vi "Read Global Message Count.vi"(8 "error in":errorcluster, 11 "Module Handle":u32) -> (0 "error out":errorcluster, 2 "Global Message Count":u32, 3 "Module Handle out":u32)   [LabVIEW 2020, in "AIM MIL-STD-1553 Hardware API.lvlib"]
uses:
  AIM MIL-STD-1553 Hardware API.lvlib
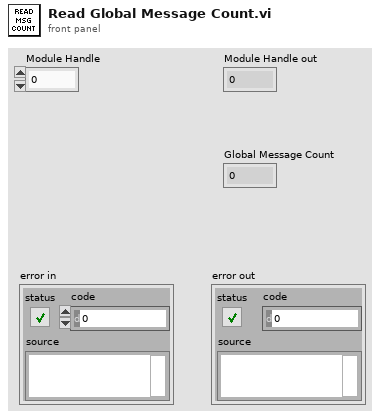
[diagram p1: front panel]
types:
  T1 = typedef "1553 All Status Counters.ctl" = cluster{"Global Message Count":u32, "Global Error Count":u32, "Primary Current Load":dbl, "Primary Average Load":dbl, "Secondary Current Load":dbl, "Secondary Average Load":dbl, "RT 1":cluster{"Active":bool, "Errors":bool, "Message Count":u32, "Error Count":u32}, "RT 2":cluster{"Active":bool, "Errors":bool, "Message Count":u32, "Error Count":u32}, "RT 3":cluster{"Active":bool, "Errors":bool, "Message Count":u32, "Error Count":u32}, "RT 4":cluster{"Active":bool, "Errors":bool, "Message Count":u32, "Error Count":u32}, "RT 5":cluster{"Active":bool, "Errors":bool, "Message Count":u32, "Error Count":u32}, "RT 6":cluster{"Active":bool, "Errors":bool, "Message Count":u32, "Error Count":u32}, "RT 7":cluster{"Active":bool, "Errors":bool, "Message Count":u32, "Error Count":u32}, "RT 8":cluster{"Active":bool, "Errors":bool, "Message Count":u32, "Error Count":u32}, "RT 9":cluster{"Active":bool, "Errors":bool, "Message Count":u32, "Error Count":u32}, "RT 10":cluster{"Active":bool, "Errors":bool, "Message Count":u32, "Error Count":u32}, "RT 11":cluster{"Active":bool, "Errors":bool, "Message Count":u32, "Error Count":u32}, "RT 12":cluster{"Active":bool, "Errors":bool, "Message Count":u32, "Error Count":u32}, "RT 13":cluster{"Active":bool, "Errors":bool, "Message Count":u32, "Error Count":u32}, "RT 14":cluster{"Active":bool, "Errors":bool, "Message Count":u32, "Error Count":u32}, "RT 15":cluster{"Active":bool, "Errors":bool, "Message Count":u32, "Error Count":u32}, "RT 16":cluster{"Active":bool, "Errors":bool, "Message Count":u32, "Error Count":u32}, "RT 17":cluster{"Active":bool, "Errors":bool, "Message Count":u32, "Error Count":u32}, "RT 18":cluster{"Active":bool, "Errors":bool, "Message Count":u32, "Error Count":u32}, "RT 19":cluster{"Active":bool, "Errors":bool, "Message Count":u32, "Error Count":u32}, "RT 20":cluster{"Active":bool, "Errors":bool, "Message Count":u32, "Error Count":u32}, "RT 21":cluster{"Active":bool, "Errors":bool, "Message Count":u32, "Error Count":u32}, "RT 22":cluster{"Active":bool, "Errors":bool, "Message Count":u32, "Error Count":u32}, "RT 23":cluster{"Active":bool, "Errors":bool, "Message Count":u32, "Error Count":u32}, "RT 24":cluster{"Active":bool, "Errors":bool, "Message Count":u32, "Error Count":u32}, "RT 25":cluster{"Active":bool, "Errors":bool, "Message Count":u32, "Error Count":u32}, "RT 26":cluster{"Active":bool, "Errors":bool, "Message Count":u32, "Error Count":u32}, "RT 27":cluster{"Active":bool, "Errors":bool, "Message Count":u32, "Error Count":u32}, "RT 28":cluster{"Active":bool, "Errors":bool, "Message Count":u32, "Error Count":u32}, "RT 29":cluster{"Active":bool, "Errors":bool, "Message Count":u32, "Error Count":u32}, "RT 30":cluster{"Active":bool, "Errors":bool, "Message Count":u32, "Error Count":u32}, "RT 31":cluster{"Active":bool, "Errors":bool, "Message Count":u32, "Error Count":u32}}
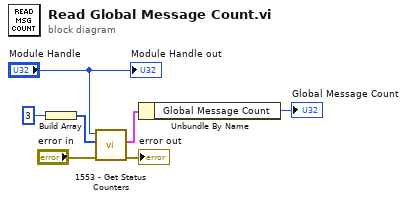
[diagram p0: block diagram]
diagram:
  n1 = Build Array(u8 3 ("RT Address (1)")) -> (w3:u8[])
  n2 = call <instrlib>:"1553 - Get Status Counters.vi"("Error In (none)"="error in", "RT Array"=w3, "Module Handle"="Module Handle") -> ("Error Out"=→"error out":errorcluster, "System Status"=w4:T1)  [unwired: 6 in, 1 out]
  n3 = Unbundle By Name(w4) -> ("Global Message Count"=→"Global Message Count":u32)
  "Module Handle out" <- "Module Handle"
